vi "StopRequest.vi"(8 "error in (no error)":errorcluster, 9 "Wait for Module to stop? (F)":bool, 11 "ModuleAdmin":refnum<class "ModuleAdmin.lvclass">) -> (0 "error out":errorcluster, 2 "Wait to Stop":bool)   [LabVIEW 2014, in "MyPluggableModule.lvlib"]
uses:
  MyPluggableModule.lvlib
  <userlib>/NIST/ModuleAdminLib/ModuleAdmin/ModuleAdmin.lvclass
  <vilib>/event_ctls.llb/usereventprio.ctl
  Arguments/Requests/clStopArgument.ctl
  clEventType.ctl
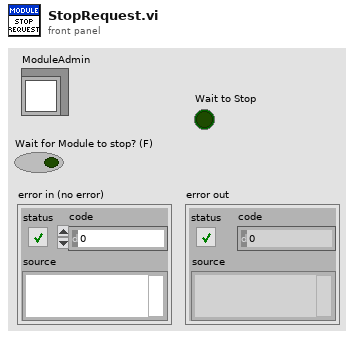
[diagram p1: front panel]
types:
  T1 = typedef "MyPluggableModule.lvlib/clRequestEvents.ctl" = cluster{"StopRequest":refnum<user-event>, "PathToINI":refnum<user-event>, " LoadPlugin":refnum<user-event>, "ShowPanel":refnum<user-event>, "PrefDlg":refnum<user-event>}
  T2 = typedef "MyPluggableModule.lvlib/clEventType.ctl" = cluster{"ModuleID":i32, "Data":variant}
  T3 = typedef "MyPluggableModule.lvlib/clStopArgument.ctl" = cluster{"Exit via Stop Module Req?":bool, "Wait for Module to stop?":bool, "ModuleAdmin":refnum<class "ModuleAdmin.lvclass">}
  T4 = typedef "usereventprio.ctl" = enum32{"high priority", "normal priority"}
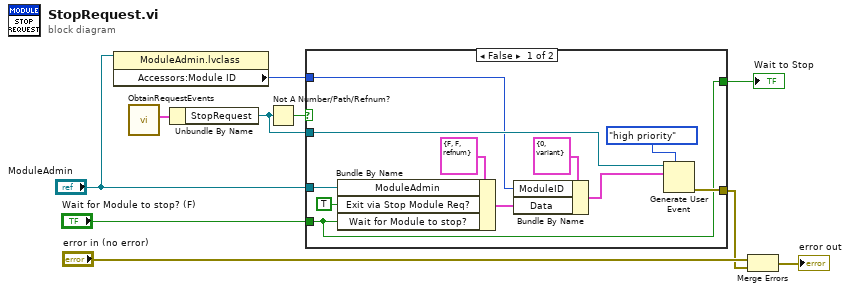
[diagram p0: block diagram]
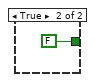
[diagram p2: hidden frame]
diagram:
  n1 = property class="ModuleAdmin.lvclass"(reference="ModuleAdmin") -> ("Accessors:Module ID"=w2:i32)  [unwired: 1 in, 2 out]
  n2 = call "ObtainRequestEvents.vi"() -> ("clRequestEvents"=w10:T1)  [unwired: 10 in, 1 out]
  n3 = Unbundle By Name(w10) -> ("StopRequest"=w8:refnum<user-event>)
  n4 = Not A Number/Path/Refnum?(number/path/refnum=w8) -> (NaN/Path/Refnum?=w9:bool)
  n5 = case shown="False" w9 {
    tunnel: w8 -> [w21 _]
    tunnel: "ModuleAdmin" -> [w14 _]
    tunnel: "Wait for Module to stop? (F)" -> [w11 _]
    tunnel: [w13 _] -> w4
    tunnel: w2 -> [w12 _]
    tunnel: [w11 FALSE] -> w1
    frame False {
      n6 = Bundle By Name(cluster=T3 {"Exit via Stop Module Req?"=FALSE, "Wait for Module to stop?"=FALSE, "ModuleAdmin"=refnum} ("Stop Argument"), "ModuleAdmin"=w14, "Exit via Stop Module Req?"=TRUE, "Wait for Module to stop?"=w11) -> (w16:T3)
      n7 = Bundle By Name(cluster=T2 {"ModuleID"=0, "Data"=variant} ("clBroadcast"), "ModuleID"=w12, "Data"=w16) -> (w15:T2)
      n8 = Generate User Event(priority (normal)=usereventprio."high priority", user event=w21, event data cluster=w15) -> (error out=w13:errorcluster)  [unwired: 1 in, 1 out]
    }
    frame True {
    }
  }
  "Wait to Stop" <- w1
  n9 = Merge Errors("error in (no error)", w4) -> (→"error out":errorcluster)
